vi "Query DA output scale.vi"(8 "error in (no error)":errorcluster, 11 "VISA resource name":refnum<visa-resource-name>) -> (0 "error out":errorcluster, 2 "output":T1, 3 "VISA resource name out":refnum<visa-resource-name>)   [LabVIEW 2009, in "SR400.lvlib"]
doc: "AM { j }\nIf j is included, the AM command sets the D/A\noutput scale. If j is absent, the D/A output scale is\nreturned.\n\nj Output scale\n0 Log (1V/decade)\n1 987######\n2 #876#####\n3 ##765####\n4 ###654###\n5 ####543##\n6 #####432#\n7 ######321"
uses:
  SR400.lvlib
  Typedefs.llb/Output Scale.ctl
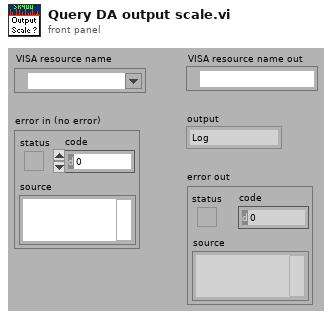
[diagram p1: front panel]
types:
  T1 = typedef "SR400.lvlib/Output Scale.ctl" = enum16{"Log", "987######", "#876#####", "##765####", "###654###", "####543##", "#####432#", "######321"}
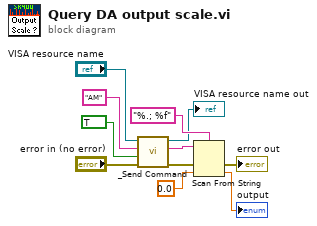
[diagram p0: block diagram]
diagram:
  n1 = call "_Send Command.vi"("error in (no error)"="error in (no error)", "Query? (F)"=TRUE, "Command"="AM" ("command"), "VISA resource name"="VISA resource name") -> ("error out"=w2:errorcluster, "Response"=w3:string, "VISA resource name out"=→"VISA resource name out":refnum<visa-resource-name>)  [unwired: 5 out]
  n2 = Scan From String(format string="%.; %f", input string=w3, error in=w2, default 1=0.0 ("default value 1")) -> (error out=→"error out":errorcluster, output 1=→"output":dbl)  [unwired: 1 in, 2 out]
